vi "Get True Owning Pane.vi"(8 "error in (no error)":errorcluster, 11 "Ctl Ref":refnum<vi>) -> (0 "error out":errorcluster, 3 "Owning Pane":refnum<vi>)   [LabVIEW 2020, in "MacroAssert.lvlib"]
doc: "Outputs the \"true owning pane\" of the control, taking into account controls within clusters."
uses:
  MacroAssert.lvlib
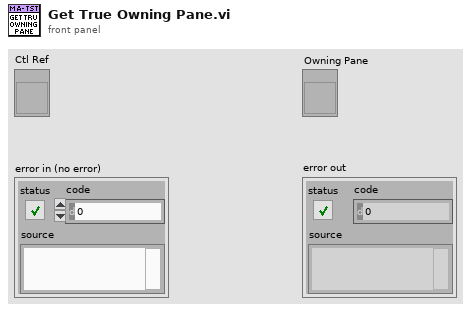
[diagram p1: front panel]
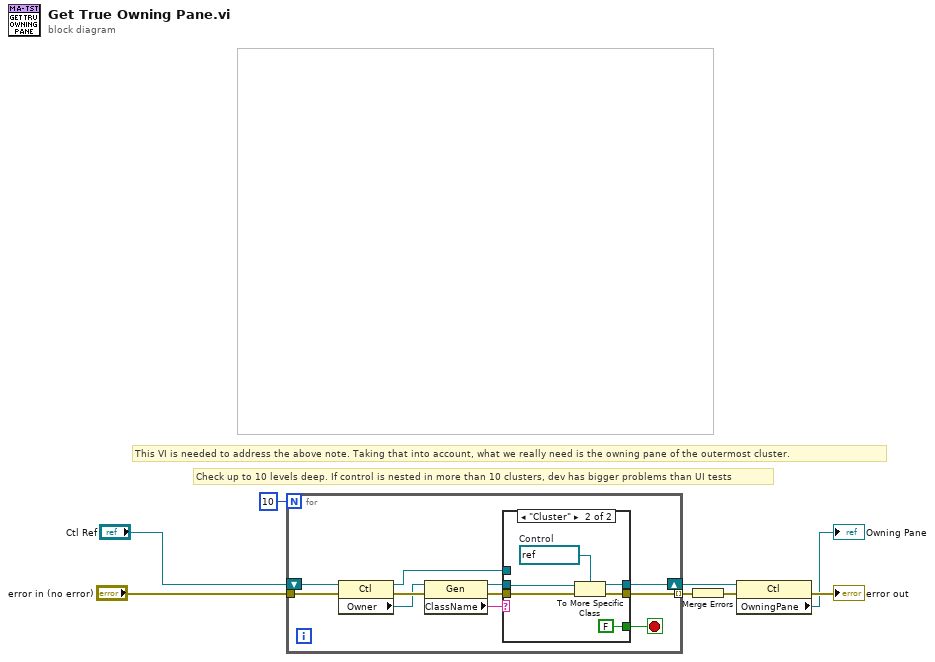
[diagram p0: block diagram]
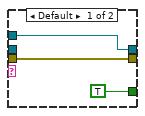
[diagram p2: hidden frame]
diagram:
  # "This VI is needed to address the above note. Taking that into account, what we really need is the owning pane of the outermost cluster."
  # "Check up to 10 levels deep. If control is nested in more than 10 clusters, dev has bigger problems than UI tests"
  n1 = for {
    N: 10 -> [_]
    tunnel: "error in (no error)" -> [w19]
    shift-right: [w12] -> w3
    shift-left: "Ctl Ref" -> [w18]
    tunnel: [w11] -> w5 mode=indexing
    stop <- w10 stop-if-true
    n2 = property class="Ctl"(reference=w18, error in=w19) -> (reference out=w9:refnum<vi>, error out=w17:errorcluster, "Owner"=w16:refnum<vi>)
    n3 = property class="Gen"(reference=w16, error in=w17) -> (reference out=w13:refnum<vi>, error out=w15:errorcluster, "ClassName"=w14:string)
    n4 = case shown="\"Cluster\"" w14 {
      tunnel: w15 -> [w21 w28]
      tunnel: w13 -> [_ w27]
      tunnel: [w20 w25] -> w12
      tunnel: [w21 w24] -> w11
      tunnel: [TRUE FALSE] -> w10
      tunnel: w9 -> [w20 _]
      frame Default {
      }
      frame "Cluster" {
        w26 = refnum<vi> refnum  # Control
        n5 = To More Specific Class(target class=w26, reference=w27, error in=w28) -> (specific class reference=w25:refnum<vi>, error out=w24:errorcluster)
      }
    }
  }
  n6 = Merge Errors(w5) -> (w4:errorcluster)
  n7 = property class="Ctl"(reference=w3, error in=w4) -> (error out=→"error out":errorcluster, "OwningPane"=→"Owning Pane":refnum<vi>)  [unwired: 1 out]
